vi "SRV_PM_Add Data to Packet Arrays.vi"(0 "Previous Packet Data":u8[](array[numeric]) format="%.0x", 5 "New Packet Data":u8[](array[numeric]) format="%.0x", 7 "Array of Packets":T1[](array[typedef]) {"Packet Data" format="%.0x"}) -> (8 "Array of Packets out":T1[](array[typedef]) {"Packet Data" format="%.0x"})   [LabVIEW 2009]
uses:
  SRV_PM_Packet.ctl
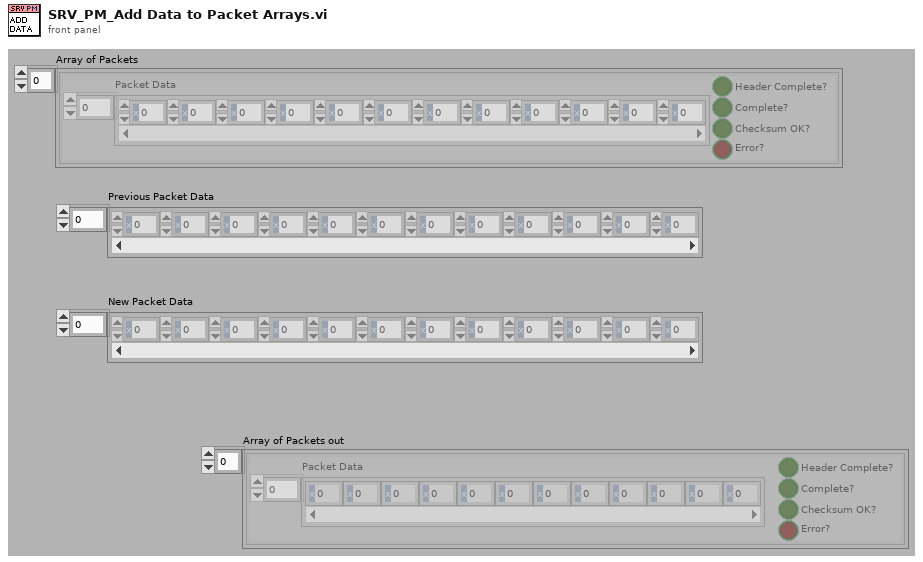
[diagram p1: front panel]
types:
  T1 = typedef "SRV_PM_Packet.ctl" = cluster{"Packet Data":u8[], "Header Complete?":bool, "Complete?":bool, "Checksum OK?":bool, "Error?":bool}
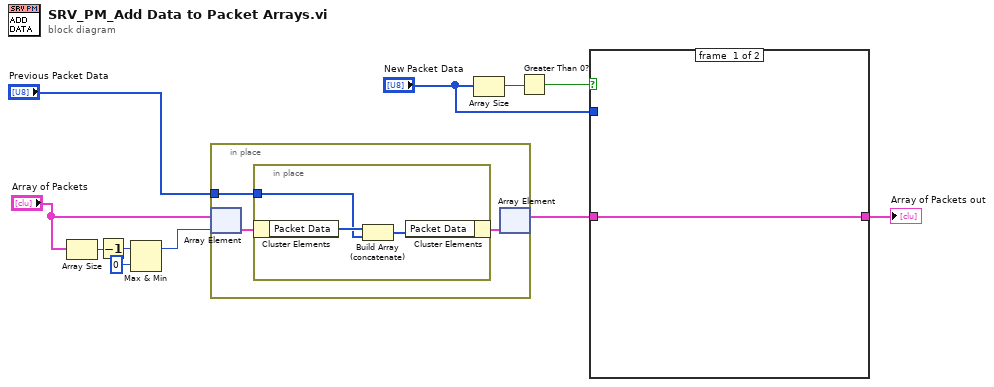
[diagram p0: block diagram]
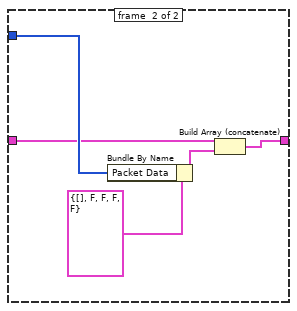
[diagram p2: hidden frame]
diagram:
  n1 = Array Size(array="Array of Packets") -> (size(s)=w9:i32)
  n2 = Decrement(x=w9) -> (x-1=w10:i32)
  n3 = Max & Min(x=w10, y=0) -> (max(x,y)=w7:i32)  [unwired: 1 out]
  n4 = in-place {
    in-place-border: "Previous Packet Data" -> [w13]
    n5 = in-place-array #1("Array of Packets", w7) -> (w14:T1)
    n6 = in-place {
      in-place-border: w13 -> [w16]
      n7 = in-place-cluster #2(w14) -> ("Packet Data"=w17:u8[])
      n8 = Build Array (concatenate)(w17, w16) -> (w15:u8[])
      n9 = in-place-cluster #2("Packet Data"=w15) -> (w12:T1)
    }
    n10 = in-place-array #1(w12) -> (w3:T1[])  [unwired: 1 out]
  }
  n11 = Array Size(array="New Packet Data") -> (size(s)=w5:i32)
  n12 = Greater Than 0?(x=w5) -> (x > 0?=w4:bool)
  n13 = case shown="False" w4 {
    tunnel: w3 -> [w18 w21]
    tunnel: [w18 w19] -> w2
    tunnel: "New Packet Data" -> [_ w22]
    frame #0 {
    }
    frame #1 {
      n14 = Bundle By Name(cluster=T1 {"Packet Data"=[], "Header Complete?"=FALSE, "Complete?"=FALSE, "Checksum OK?"=FALSE, "Error?"=FALSE} ("Packet"), "Packet Data"=w22) -> (w20:T1)
      n15 = Build Array (concatenate)(w21, w20) -> (w19:T1[])
    }
  }
  "Array of Packets out" <- w2
